vi "생산자 소비자 (delay 적용).vi"() -> ()   [LabVIEW 2014]
panel:
  out "웨이브폼 차트":dbl(graph)
  out "메시지":string
  in  "확인 버튼":bool
  in  "정지":bool
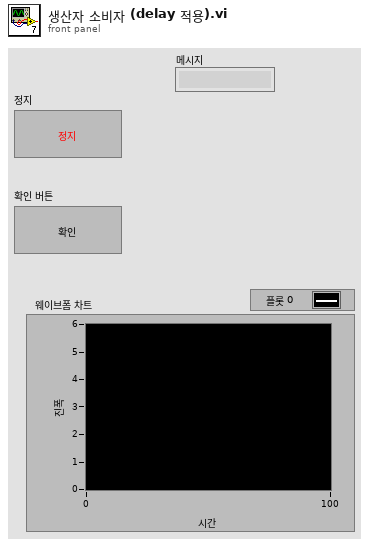
[diagram p1: front panel]
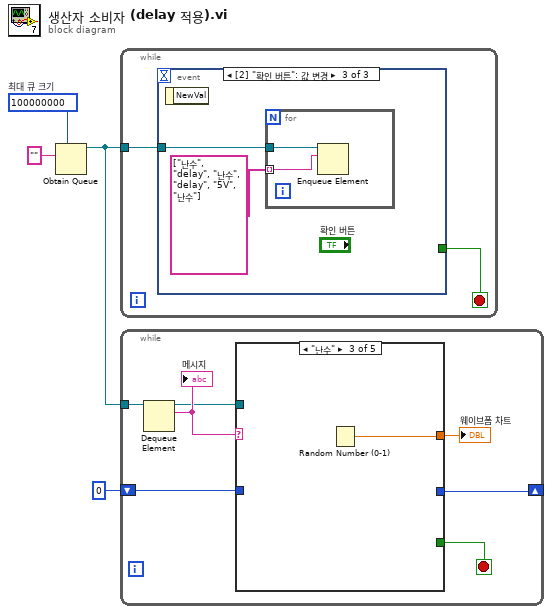
[diagram p0: block diagram]
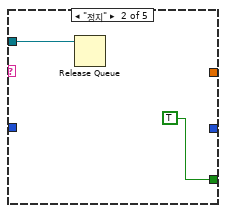
[diagram p3: hidden frame]
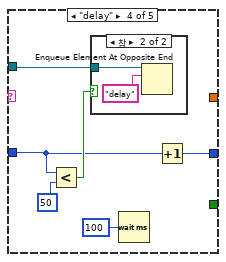
[diagram p4: hidden frame]
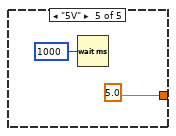
[diagram p6: hidden frame]
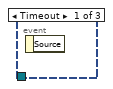
[diagram p7: hidden frame]
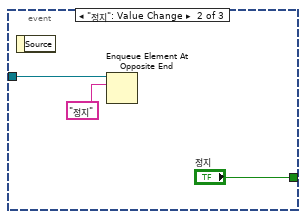
[diagram p8: hidden frame]
diagram:
  w2 = 100000000  # 최대 큐 크기
  n1 = Obtain Queue(max queue size (-1, unlimited)=w2, element data type="") -> (queue out=w1:refnum<queue>)  [unwired: 3 in, 2 out]
  n2 = while {
    tunnel: w1 -> [w5]
    stop <- w6 stop-if-true
    n3 = event shown="[2] \"확인 버튼\": 값 변경" {
      selector: _ -> [_ _ _]
      dyn-events: _ -> [_ _ _]
      timeout: _ -> [_ _ _]
      tunnel: [_ "정지" _] -> w6
      tunnel: w5 -> [_ w7 w11]
      event Timeout {
        n4 = event-data() -> ()  [unwired: 1 in, 1 out]
      }
      event "정지": Value Change {
        n5 = event-data() -> ()  [unwired: 1 in, 1 out]
        n6 = Enqueue Element At Opposite End(queue=w7, element="정지" ("원소")) -> ()  [unwired: 2 in, 3 out]
      }
      event "확인 버튼": Value Change {
        n7 = event-data() -> ()  [unwired: 1 in, 1 out]
        n8 = for {
          tunnel: w11 -> [w13]
          tunnel: string[] ["난수", "delay", "난수", "delay", "5V", "난수"] -> [w12] mode=indexing
          n9 = Enqueue Element(queue=w13, element=w12) -> ()  [unwired: 2 in, 3 out]
        }
      }
    }
  }
  n10 = while {
    tunnel: w1 -> [w20]
    shift-right: [w15] -> _
    shift-left: 0 -> [w16]
    stop <- w18 stop-if-true
    n11 = Dequeue Element(queue=w20) -> (queue out=w14:refnum<queue>, element=w19:string)  [unwired: 2 in, 2 out]
    "메시지" <- w19
    n12 = case shown="\"난수\"" w19 {
      tunnel: [_ TRUE _ _ _] -> w18
      tunnel: [_ _ w23 _ 5.0] -> w17
      tunnel: w14 -> [_ w21 _ w27 _]
      tunnel: w16 -> [_ _ _ w24 _]
      tunnel: [_ _ _ w29 _] -> w15
      frame "거짓", Default {
      }
      frame "정지" {
        n13 = Release Queue(queue=w21) -> ()  [unwired: 2 in, 3 out]
      }
      frame "난수" {
        n14 = Random Number (0-1)() -> (number: 0 to 1=w23:dbl)
      }
      frame "delay" {
        n15 = Less?(x=w24, y=50) -> (x < y?=w26:bool)
        n16 = case shown="참" w26 {
          tunnel: w27 -> [_ w31]
          frame False {
          }
          frame True {
            n17 = Enqueue Element At Opposite End(queue=w31, element="delay" ("원소")) -> ()  [unwired: 2 in, 3 out]
          }
        }
        n18 = Wait (ms)(milliseconds to wait=u32 100 ("대기 시간(ms)")) -> ()  [unwired: 1 out]
        n19 = Increment(x=w24) -> (x+1=w29:i32)
      }
      frame "5V" {
        n20 = Wait (ms)(milliseconds to wait=u32 1000 ("대기 시간(ms)")) -> ()  [unwired: 1 out]
      }
    }
    "웨이브폼 차트" <- w17
  }
